vi "GetGXMLCfgVolt.vi"(8 "error in (no error)":errorcluster, 11 "Voltage in":refnum<class "Voltage.lvclass">) -> (0 "error out":errorcluster, 2 "Voltage Cfg":T1, 3 "Voltage out":refnum<class "Voltage.lvclass">)   [LabVIEW 2012, in "Measurement Channels.lvlib" / "Voltage.lvclass"]
uses:
  Voltage.lvclass
  VoltProps_TD.ctl
  Voltage.lvclass/Voltage.ctl
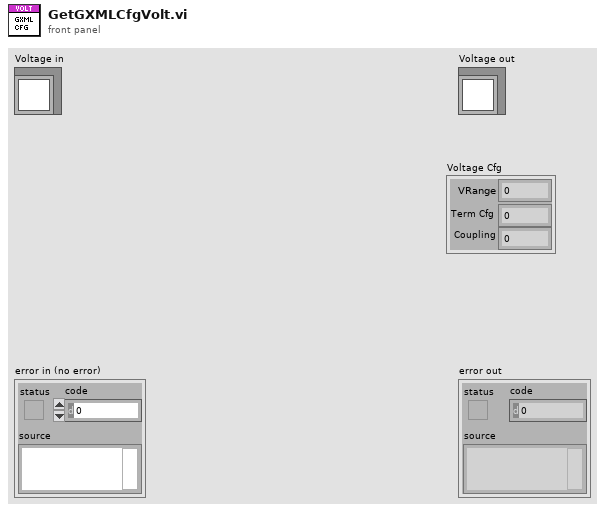
[diagram p1: front panel]
types:
  T1 = typedef "Measurement Channels.lvlib/Voltage.lvclass/VoltProps_TD.ctl" = cluster{"VRange":dbl, "Term Cfg":u16, "Coupling":u16}
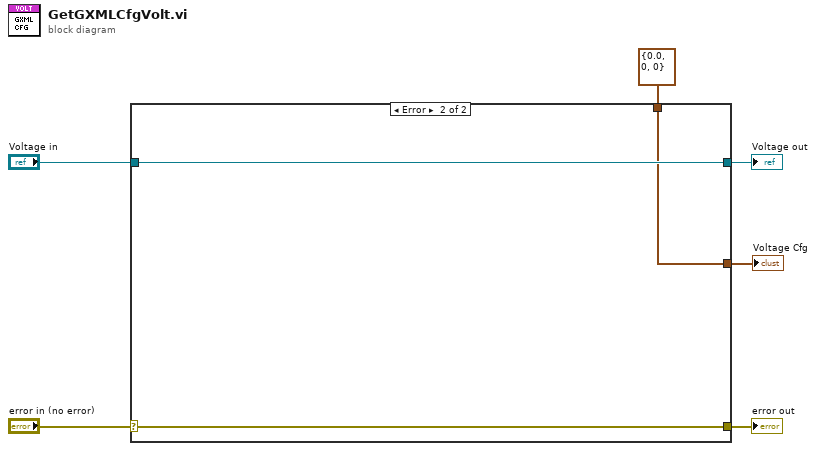
[diagram p0: block diagram]
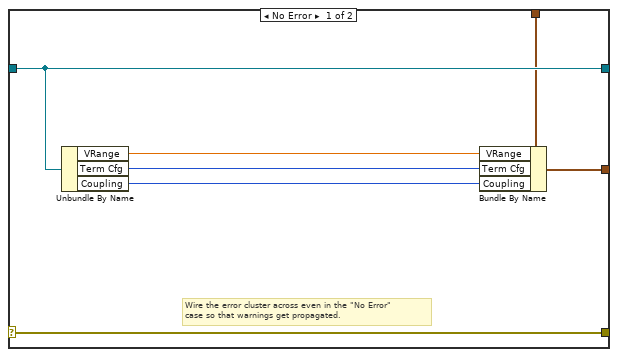
[diagram p2: hidden frame]
diagram:
  n1 = case shown="Error" "error in (no error)" {
    selector: "error in (no error)" -> [w13 w16]
    tunnel: [w13 w16] -> w5
    tunnel: [w12 w15] -> w3
    tunnel: "Voltage in" -> [w12 w15]
    tunnel: T1 {"VRange"=0.0, "Term Cfg"=0, "Coupling"=0} ("VoltChanCfg") -> [w8 w14]
    tunnel: [w7 w14] -> w1
    frame No Error {
      # "Wire the error cluster across even in the \"No Error\"\ncase so that warnings get propagated."
      n2 = Unbundle By Name(w12) -> ("VRange"=w11:dbl, "Term Cfg"=w10:u16, "Coupling"=w9:u16)
      n3 = Bundle By Name(cluster=w8, "VRange"=w11, "Term Cfg"=w10, "Coupling"=w9) -> (w7:T1)
    }
    frame Error {
    }
  }
  "error out" <- w5
  "Voltage out" <- w3
  "Voltage Cfg" <- w1
